vi "DSF.Engine.Framework.Start.vi"(8 "error in (no error)":errorcluster, 11 "Framework in":refnum<class "DSF.Engine.Framework.lvclass">) -> (0 "error out":errorcluster, 3 "Framework out":refnum<class "DSF.Engine.Framework.lvclass">)   [LabVIEW 2017, in "Data Sharing Framework Engine.lvlib" / "DSF.Engine.Framework.lvclass"]
uses:
  DSF.Engine.Framework.lvclass
  DSF.Engine.Framework.lvclass/DSF.Engine.Framework.ctl
  Plugin/DSF.Engine.Plugin.lvclass
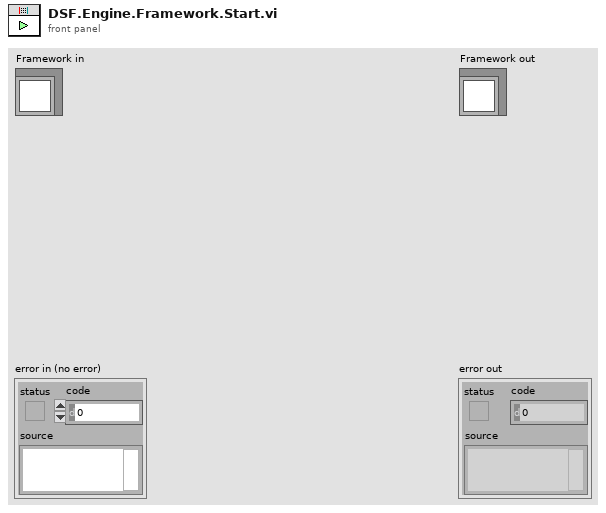
[diagram p1: front panel]
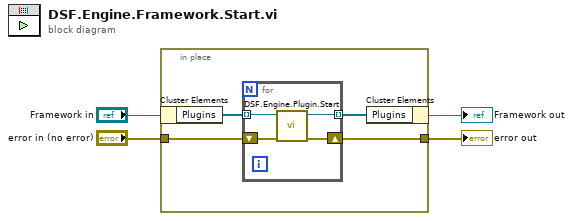
[diagram p0: block diagram]
diagram:
  n1 = in-place {
    in-place-border: "error in (no error)" -> [w8]
    in-place-border: [w7] -> w3
    n2 = in-place-cluster #1("Framework in") -> ("Plugins"=w6:refnum<class "DSF.Engine.Plugin.lvclass">[])
    n3 = for {
      tunnel: w6 -> [w12] mode=indexing
      tunnel: [w11] -> w5 mode=indexing
      shift-right: [w10] -> w7
      shift-left: w8 -> [w9]
      n4 = call "DSF.Engine.Plugin.Start.vi"("error in (no error)"=w9, "Plugin in"=w12) -> ("error out"=w10:errorcluster, "Plugin out"=w11:refnum<class "DSF.Engine.Plugin.lvclass">)  [unwired: 8 in]
    }
    n5 = in-place-cluster #1("Plugins"=w5) -> (→"Framework out":refnum<class "DSF.Engine.Framework.lvclass">)
  }
  "error out" <- w3
